vi "OVP-OCP set(on-off).vi"(4 "OCP":enum16{"ON", "OFF"}(ring), 6 "OVP":enum16{"ON", "OFF"}(ring), 7 "Channel  (1: CH1)":u16(ring)=1 items=["CH1"=1, "CH2"=2, "CH3"=3, "CH4"=4], 8 "error in (no error)":errorcluster, 11 "VISA resource in":refnum<visa-resource-name>) -> (0 "error out":errorcluster, 3 "VISA resource name out":refnum<visa-resource-name>)   [LabVIEW 2020, in "GPP.lvlib"]
uses:
  GPP.lvlib
  Function/VISA_COMMON.ctl
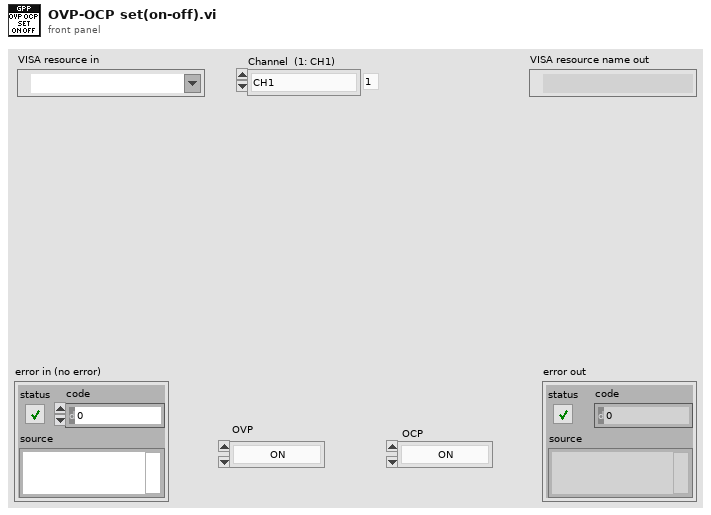
[diagram p1: front panel]
types:
  T1 = typedef "GPP.lvlib/VISA_COMMON.ctl" = enum16{"Initial", "Write CMD", "Read Result", "Read History", "Close"}
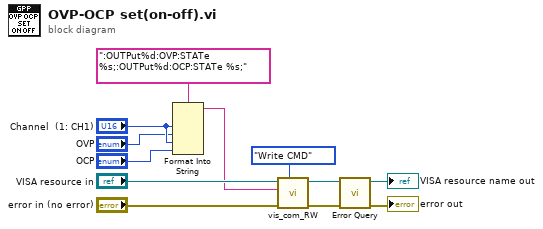
[diagram p0: block diagram]
diagram:
  n1 = Format Into String(format string=":OUTPut%d:OVP:STATe %s;:OUTPut%d:OCP:STATe %s;", "Channel  (1: CH1)", "OVP", "Channel  (1: CH1)", "OCP") -> (resulting string=w5:string)  [unwired: 2 in, 1 out]
  n2 = call "vis_com_RW.vi"("Funciton"=VISA_COMMON."Write CMD", "error in (no error)"="error in (no error)", "CMD String"=w5, "VISA resource in"="VISA resource in") -> ("error out"=w11:errorcluster, "VISA resource out"=w12:refnum<visa-resource-name>)  [unwired: 5 in, 1 out]
  n3 = call "Error Query.vi"("error in (no error)"=w11, "VISA resource name"=w12) -> ("error out"=→"error out":errorcluster, "VISA resource name out"=→"VISA resource name out":refnum<visa-resource-name>)  [unwired: 6 in, 2 out]
